vi "Last_Years_Setups.vi"(1 "Setup File Type":T1) -> (0 "Directory":path)   [LabVIEW 2011]
uses:
  Setup_Filetype.ctl
  Globals/Constants_global.vi
  Globals/Preference_global.vi
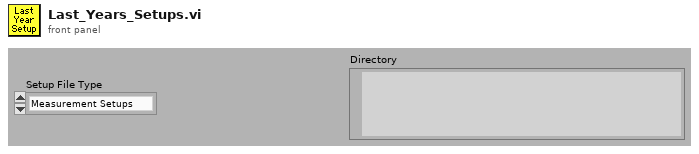
[diagram p1: front panel]
types:
  T1 = typedef "Setup_Filetype.ctl" = enum16{"Measurement Setups", "Calibration Setups", "General", "Results File Plotter Setups", "Speed Calib Tweaks"}
  T2 = typedef "LVDateTimeRec.ctl" = cluster{"fractional second":dbl, "second":i32, "minute":i32, "hour":i32, "day of month":i32, "month":i32, "year":i32, "day of week":i32, "day of year":i32, "DST":i32}
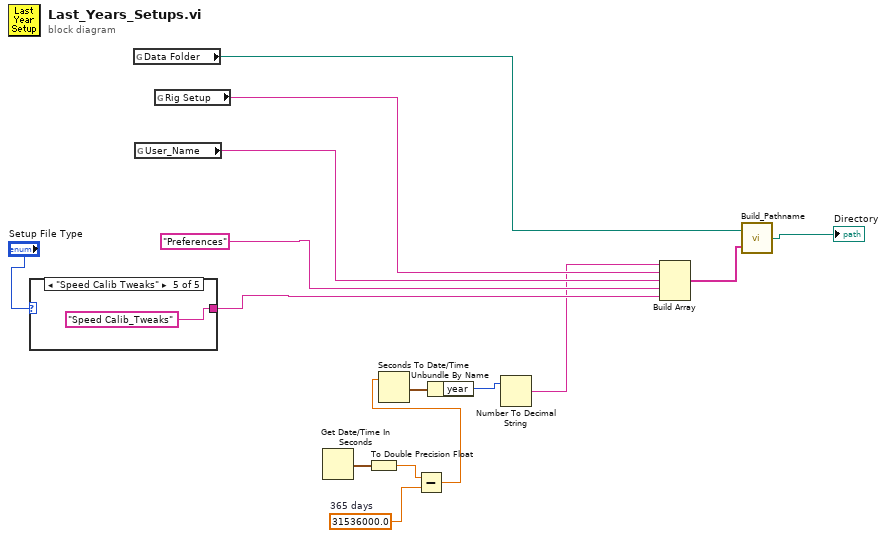
[diagram p0: block diagram]
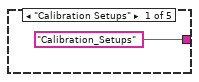
[diagram p2: hidden frame]
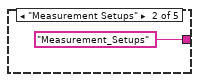
[diagram p3: hidden frame]
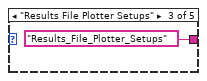
[diagram p4: hidden frame]
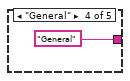
[diagram p5: hidden frame]
diagram:
  w6 = 31536000.0  # 365 days
  n1 = case shown="\"Speed Calib Tweaks\"" "Setup File Type" {
    tunnel: ["Calibration_Setups" "Measurement_Setups" "Results_File_Plotter_Setups" "General" ("name or relative path") "Speed Calib_Tweaks" ("name or relative path")] -> w10
    frame "Calibration Setups" {
    }
    frame "Measurement Setups" {
    }
    frame "Results File Plotter Setups" {
    }
    frame "General" {
    }
    frame "Speed Calib Tweaks" {
    }
  }
  n2 = global read "Constants_global.vi" "Data Folder"() -> (w15:path)
  n3 = global read "Preference_global.vi" "User_Name"() -> (w13:string)
  n4 = global read "Preference_global.vi" "Rig Setup"() -> (w14:string)
  n5 = Get Date/Time In Seconds() -> (seconds since 1Jan1904=w7:timestamp)
  n6 = To Double Precision Float(number=w7) -> (double precision float=w8:dbl)
  n7 = Subtract(x=w8, y=w6) -> (x-y=w3:dbl)
  n8 = Seconds To Date/Time(time stamp (now)=w3) -> (date time rec=w5:T2)  [unwired: 1 out]
  n9 = Unbundle By Name(w5) -> ("year"=w4:i32)
  n10 = Number To Decimal String(number=w4) -> (decimal integer string=w2:string)  [unwired: 1 out]
  n11 = Build Array(w2, w14, w13, "Preferences" ("name or relative path"), w10) -> (w9:string[])
  n12 = call "Build_Pathname.vi"("PathElements"=w9, "PathnameIn"=w15) -> ("AppendedPath"=→"Directory":path)
